vi "ParserStringSemicolon(SubVI).vi"(1 "value array":string) -> (0 "Array":string[](array[string]))   [LabVIEW 2018]
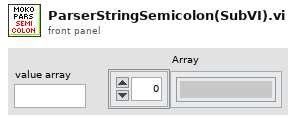
[diagram p1: front panel]
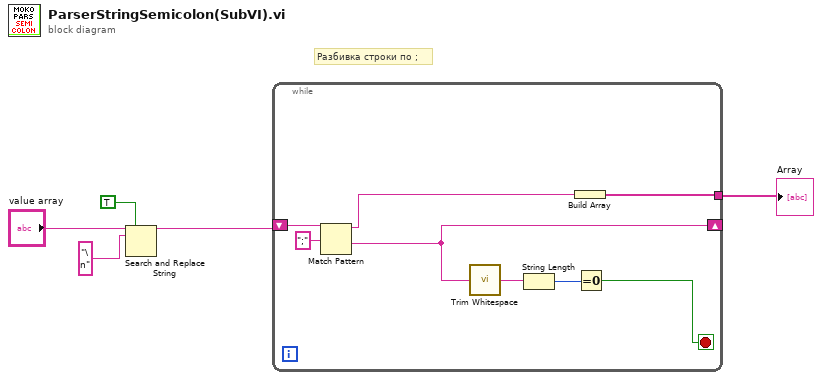
[diagram p0: block diagram]
diagram:
  # "Разбивка строки по ;"
  n1 = Search and Replace String(replace all?=TRUE ("replace all? (F)"), input string="value array", search string="\n") -> (result string=w2:string)  [unwired: 5 in, 3 out]
  n2 = while {
    shift-right: [w7] -> _
    shift-left: w2 -> [w13]
    tunnel: [w8] -> w1
    stop <- w10 stop-if-true
    n3 = Match Pattern(string=w13, regular expression=";") -> (before substring=w9:string, after substring=w7:string)  [unwired: 1 in, 2 out]
    n4 = call <vilib>:"Trim Whitespace.vi"("string"=w7) -> ("trimmed string"=w6:string)  [unwired: 1 in]
    n5 = String Length(string=w6) -> (length=w11:i32)
    n6 = Build Array(w9) -> (w8:string[])
    n7 = Equal To 0?(x=w11) -> (x = 0?=w10:bool)
  }
  "Array" <- w1
